vi "FieldDisp_Element_Prepare.vi"(5 "Element File Name":string, 7 "Element Picture Ref":refnum<vi>, 8 "error in (no error)":errorcluster, 9 "Field Height Ft":dbl=27.0, 10 "Field Width Ft":dbl=54.0, 11 "Field Picture Ref":refnum<vi>) -> (0 "error out":errorcluster, 3 "Field Element Info":T1)   [LabVIEW 2019, in "Trajectory_Library.lvlib"]
doc: "Prepare a field element (robot, game piece, etc.) for display on a field. This routine opens the image file and prepares the image for display, movement, and rotation.\n\nImage files can be PNG, BMP, or JPG.\n\nInputs:\n - Element File Name -- String -- File name of element to display. Relative paths start in the root directory of the application.\n - Element Picture Ref -- Picture Reference -- Reference to the control used to display the field element.\n - Field Picture Ref -- Picture Reference -- Reference to the control used to display the field.\n - Field Width -- double -- Width of the field (feet). This is used to initialize element positioning.\n - Field Height -- double -- Height of the field (feet). This is used to initialize element positioning.\n - Error in -- error cluster -- input error. Often used to sequence VIs.\n\nOutputs:\n - Field Element Info -- cluster -- Contains information used for display of element.\n - Error out -- error cluster -- contains error information."
uses:
  Trajectory_Library.lvlib
  TypeDef/FieldDisp_FieldElement.ctl
  <vilib>/Utility/miscctls.llb/LVBoundsTypeDef.ctl
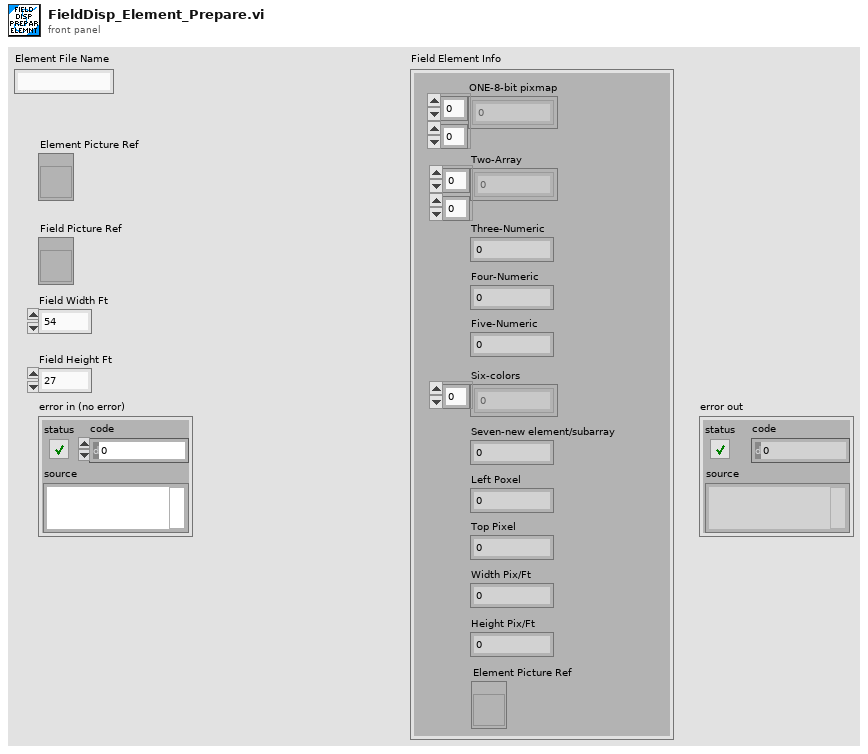
[diagram p1: front panel]
types:
  T1 = typedef "Trajectory_Library.lvlib/FieldDisp_FieldElement.ctl" = cluster{"ONE-8-bit pixmap":u8[][], "Two-Array":cdb[][], "Three-Numeric":i32, "Four-Numeric":i32, "Five-Numeric":cdb, "Six-colors":u32[], "Seven-new element/subarray":u32, "Left Poxel":dbl, "Top Pixel":dbl, "Width Pix/Ft":dbl, "Height Pix/Ft":dbl, "Element Picture Ref":refnum<vi>}
  T2 = typedef "LVBoundsTypeDef.ctl" = cluster{"Width":u32, "Height":u32}
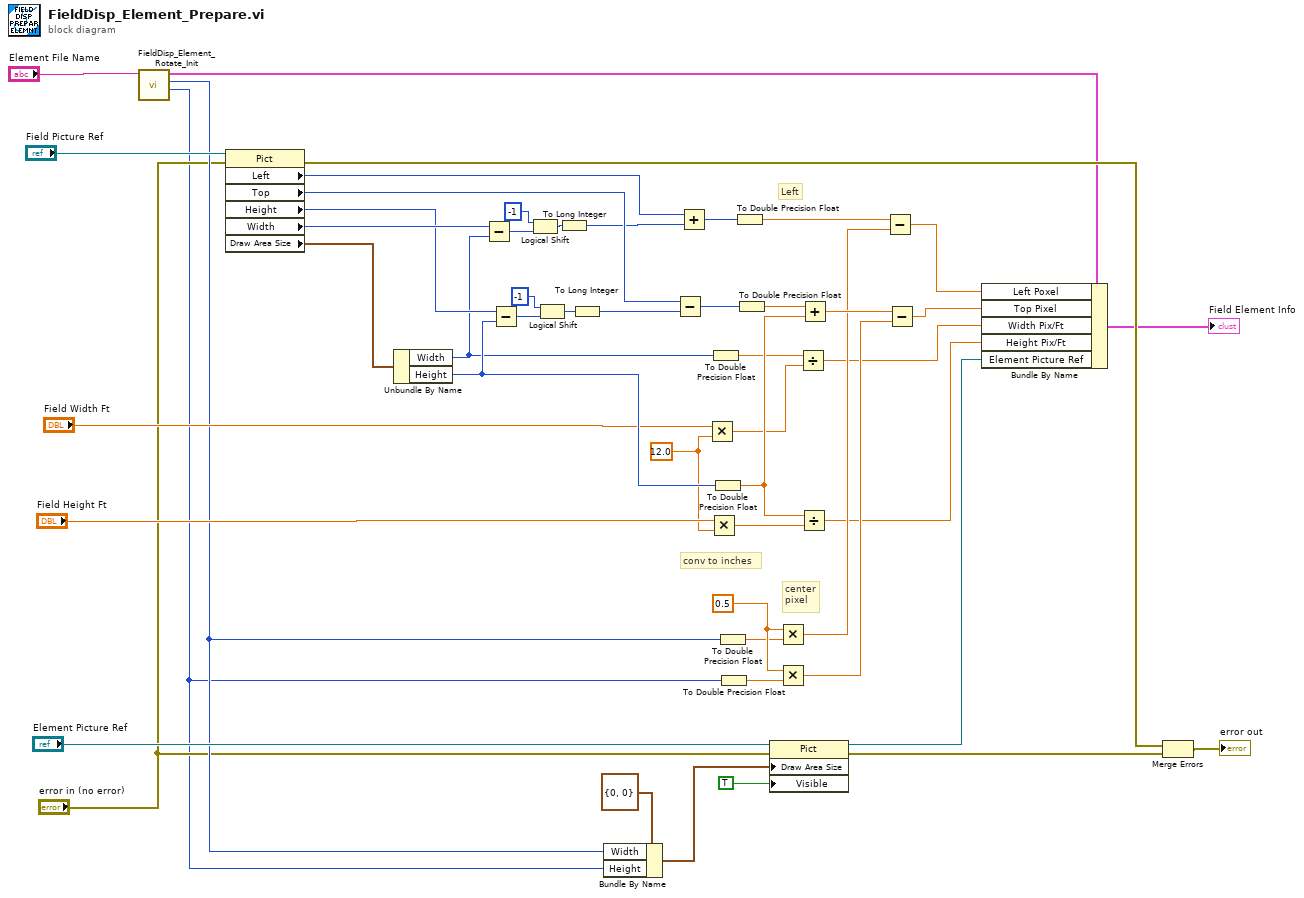
[diagram p0: block diagram]
diagram:
  w29 = 0.5
  w19 = 12.0 ("y")
  # "Left"
  # "center\npixel"
  # "conv to inches"
  n1 = call "FieldDisp_Element_Rotate_Init.vi"("Picture FIle Name"="Element File Name") -> ("Height"=w8:i16, "Width"=w13:i16, "RotatedPictureInfo"=w7:T1)  [unwired: 7 in, 1 out]
  n2 = property class="Pict"(reference="Field Picture Ref", error in="error in (no error)") -> (error out=w10:errorcluster, "Left"=w47:i32, "Top"=w48:i32, "Height"=w49:u32, "Width"=w50:u32, "Draw Area Size"=w51:T2)  [unwired: 1 out]
  n3 = Unbundle By Name(w51) -> ("Width"=w34:u32, "Height"=w38:u32)
  n4 = Subtract(x=w50, y=w34) -> (x-y=w35:u32)
  n5 = Subtract(x=w49, y=w38) -> (x-y=w37:u32)
  n6 = Logical Shift(y=i16 -1, x=w35) -> (x << y=w42:u32)
  n7 = Logical Shift(y=i16 -1, x=w37) -> (x << y=w44:u32)
  n8 = To Long Integer(number=w42) -> (32bit integer=w43:i32)
  n9 = To Long Integer(number=w44) -> (32bit integer=w45:i32)
  n10 = Bundle By Name(cluster=T2 {"Width"=0, "Height"=0} ("Draw Area Size"), "Width"=w13, "Height"=w8) -> (w16:T2)
  n11 = Subtract(x=w48, y=w45) -> (x-y=w39:i32)
  n12 = Add(x=w47, y=w43) -> (x+y=w40:i32)
  n13 = Multiply(x="Field Width Ft", y=w19) -> (x*y=w24:dbl)
  n14 = Multiply(x="Field Height Ft", y=w19) -> (x*y=w26:dbl)
  n15 = To Double Precision Float(number=w34) -> (double precision float=w23:dbl)
  n16 = To Double Precision Float(number=w38) -> (double precision float=w25:dbl)
  n17 = To Double Precision Float(number=w13) -> (double precision float=w27:dbl)
  n18 = To Double Precision Float(number=w8) -> (double precision float=w28:dbl)
  n19 = To Double Precision Float(number=w40) -> (double precision float=w30:dbl)
  n20 = To Double Precision Float(number=w39) -> (double precision float=w22:dbl)
  n21 = property class="Pict"(reference="Element Picture Ref", error in="error in (no error)", "Draw Area Size"=w16, "Visible"=TRUE) -> (reference out=w1:refnum<vi>, error out=w9:errorcluster)
  n22 = Multiply(x=w29, y=w27) -> (x*y=w31:dbl)
  n23 = Multiply(x=w29, y=w28) -> (x*y=w33:dbl)
  n24 = Divide(x=w23, y=w24) -> (x/y=w3:dbl)
  n25 = Divide(x=w25, y=w26) -> (x/y=w2:dbl)
  n26 = Add(x=w22, y=w25) -> (x+y=w32:dbl)
  n27 = Subtract(x=w30, y=w31) -> (x-y=w5:dbl)
  n28 = Subtract(x=w32, y=w33) -> (x-y=w4:dbl)
  n29 = Bundle By Name(cluster=w7, "Left Poxel"=w5, "Top Pixel"=w4, "Width Pix/Ft"=w3, "Height Pix/Ft"=w2, "Element Picture Ref"=w1) -> (→"Field Element Info":T1)
  n30 = Merge Errors(w10, w9) -> (→"error out":errorcluster)
